vi "LiveCapture.vi"(8 "error in (no error)":errorcluster, 11 "OpenCVCam in":refnum<class "OpenCVCam.lvclass">) -> (0 "error out":errorcluster, 3 "OpenCVCam out":refnum<class "OpenCVCam.lvclass">)   [LabVIEW 2021, in "OpenCVCam.lvclass"]
uses:
  OpenCVCam.lvclass
  C:/Localdata/Projects/TriekselSoft/TriekselsoftApplicationFramework/Source/.Externals/Library_YAF/YActor/YActor.lvclass
  .Externals/Library_YAF/YActor/ExeCmd_async.vi
  .Externals/Library_YAF/YActor/YActor.lvclass
  C:/Localdata/Projects/TriekselSoft/TriekselsoftApplicationFramework/Source/.Externals/Library_YAF/YAFTAF/YAFTAF.lvclass
  C:/Localdata/Projects/TriekselSoft/TriekselsoftApplicationFramework/Source/.Externals/Interface_UserInterface_IFrontPanel/IFrontPanel/IFrontPanel.lvclass
  C:/Localdata/Projects/TriekselSoft/TriekselsoftApplicationFramework/Source/IInterface/IInterface.lvclass
  C:/Localdata/Projects/TriekselSoft/TriekselsoftApplicationFramework/Source/.Externals/Interface_Object_ICreateDestroy/ICreateDestroy/ICreateDestroy.lvclass
  C:/Localdata/Projects/TriekselSoft/TriekselsoftApplicationFramework/Source/.Externals/Interface_Object_IPersistentData/IPersistentData/IPersistentData.lvclass
  C:/Localdata/Projects/TriekselSoft/TriekselsoftApplicationFramework/Source/.Externals/Interface_TAF_ITAFObject/ITAFObject/ITAFObject.lvclass
  C:/Localdata/Projects/TriekselSoft/TriekselsoftApplicationFramework/Source/YAFTAFObjects/OpenCVCam/OpenCVCam.lvclass
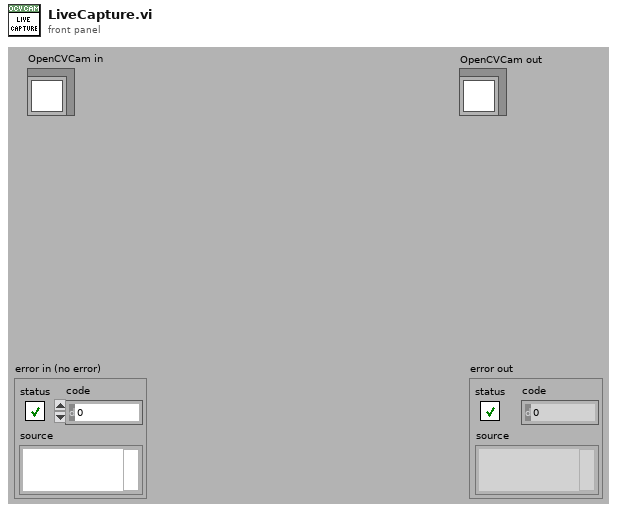
[diagram p1: front panel]
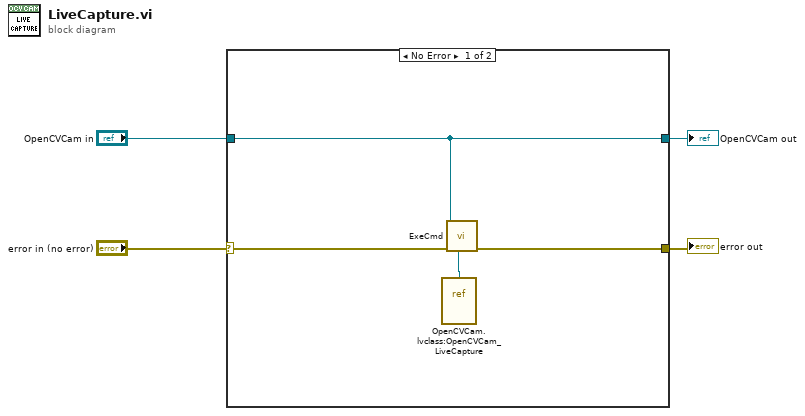
[diagram p0: block diagram]
diagram:
  n1 = case shown="No Error" "error in (no error)" {
    selector: "error in (no error)" -> [w7 w10]
    tunnel: [w5 w10] -> w3
    tunnel: [w6 w9] -> w1
    tunnel: "OpenCVCam in" -> [w6 w9]
    frame No Error {
      n2 = vi-ref "OpenCVCam.lvclass:OpenCVCam_LiveCapture.vi"() -> (w8:refnum<vi>)
      n3 = call-poly "ExeCmd.vi"("CmdVIRef"=w8, "ErrorIn"=w7, "YActor in"=w6) -> ("ErrorOut"=w5:errorcluster)  [unwired: 8 in]
    }
    frame Error {
    }
  }
  "error out" <- w3
  "OpenCVCam out" <- w1
